vi "Strings2.vi"() -> ()   [LabVIEW 2020]
uses:
  <vilib>/regexp/Match Regular Expression.xnode
panel:
  out "date/time string":string
  out "after match":string
  out "before match":string
  in  "regular expression":string
  in  "input string":string
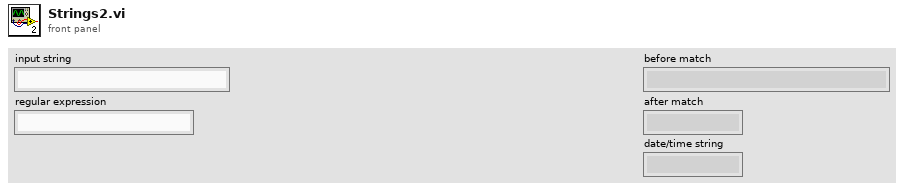
[diagram p1: front panel]
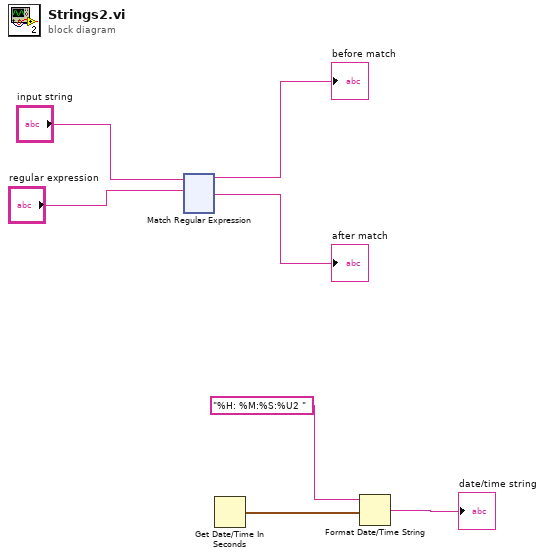
[diagram p0: block diagram]
diagram:
  n1 = xnode "Match Regular Expression"("input string"="input string", "regular expression"="regular expression") -> ("before match"=→"before match":string, "after match"=→"after match":string)  [unwired: 4 in, 3 out]
  n2 = Get Date/Time In Seconds() -> (seconds since 1Jan1904=w3:timestamp)
  n3 = Format Date/Time String(time format string (%c)="%H: %M:%S:%U2 ", seconds (now)=w3) -> (date/time string=→"date/time string":string)  [unwired: 1 in]
